vi "Test Viewer.vi"() -> ()   [LabVIEW 2016]
panel:
  out "XY Graph":cluster{"Y":dbl[], "Y":dbl[]}(graph)
  in  "channels":string[](array[string])=["Field (Resampled)", "U X (Resampled)", "U Y (Resampled)"]
  in  "group":string="p"
  in  "File Path Control":path=path "\\\\eden\\NHMFLDATA/Data/cell1daq/February_2017/021017/p002_021017.tdms"
  out "Waveform Graph":waveform(dbl)[](graph)
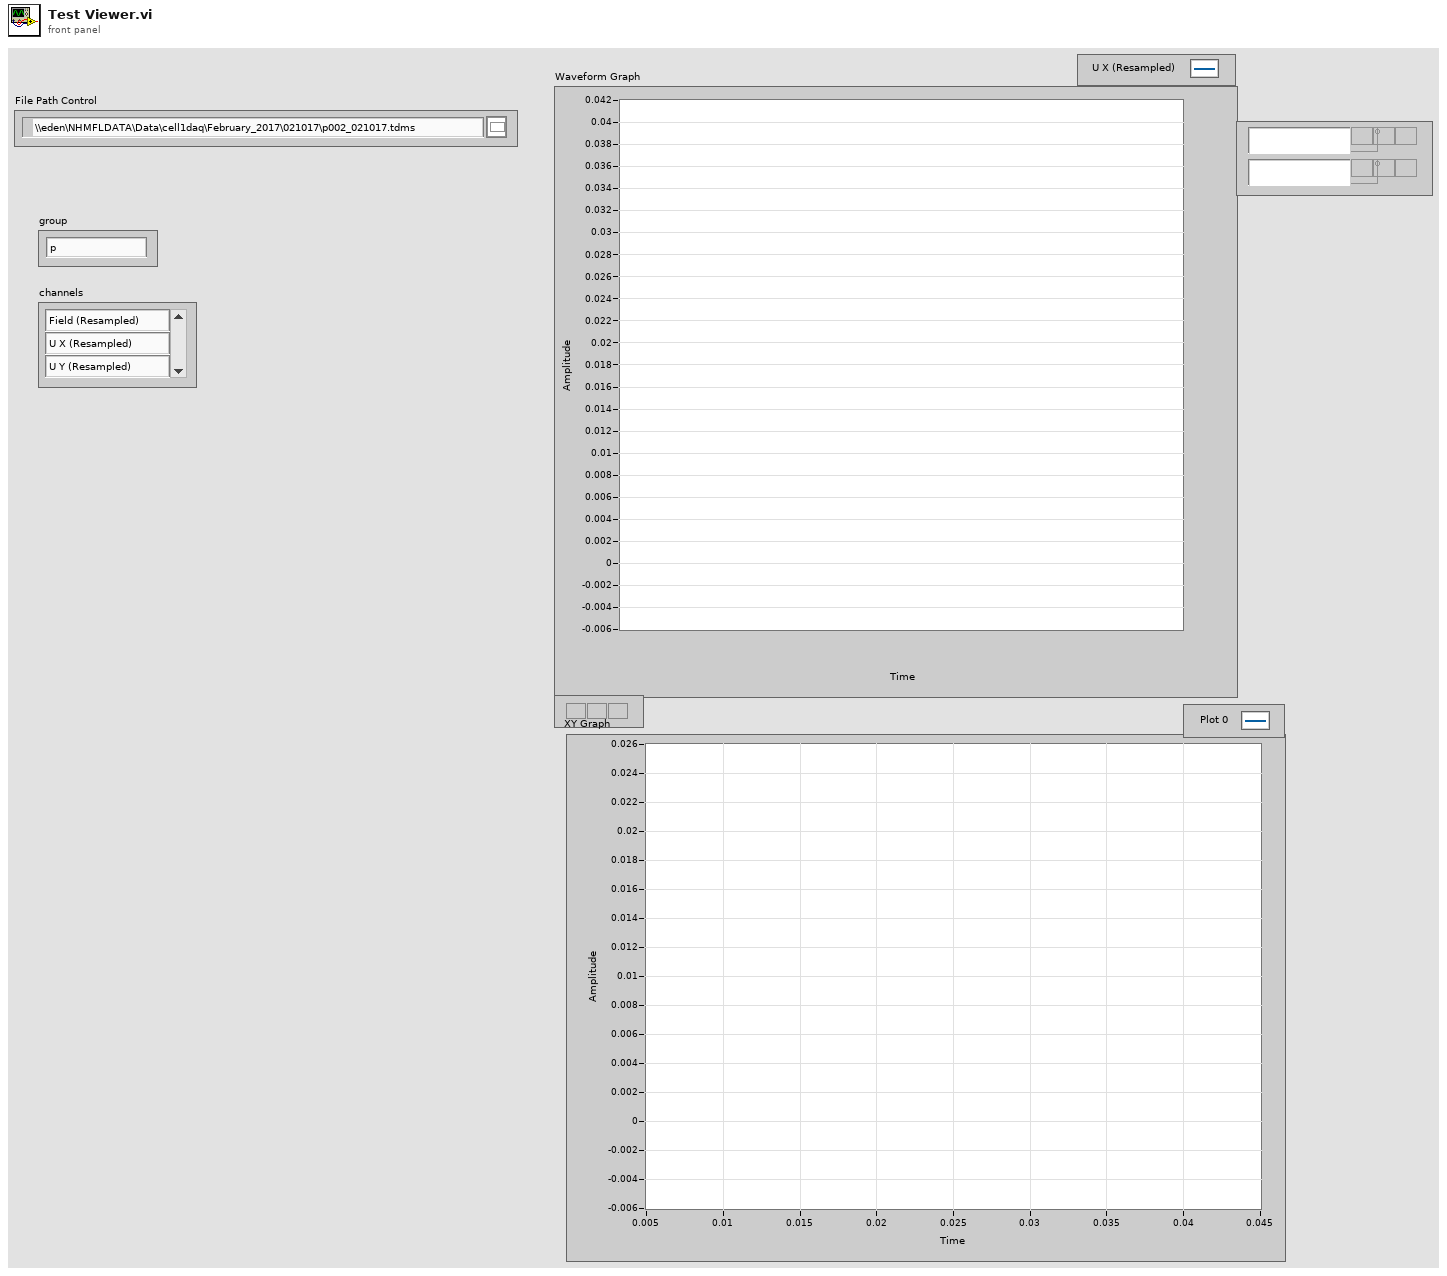
[diagram p1: front panel]
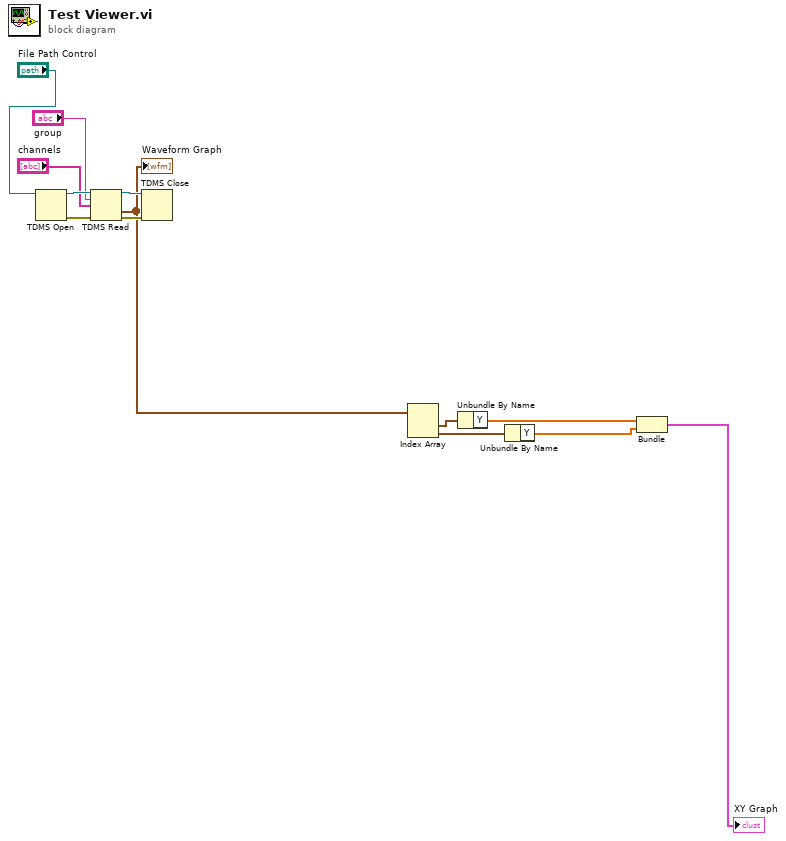
[diagram p0: block diagram]
diagram:
  n1 = TDMS Open(11:"File Path Control") -> (0:w10:errorcluster, 3:w13:refnum<k34>)  [unwired: 6 in]
  n2 = TDMS Read(0:w13, 5:"group", 7:"channels", 11:w10) -> (4:w12:refnum<k34>, 10:w6:waveform(dbl)[], 15:w11:errorcluster)  [unwired: 4 in, 3 out]
  "Waveform Graph" <- w6
  n3 = TDMS Close(8:w11, 11:w12) -> ()  [unwired: 2 out]
  n4 = Index Array(array=w6) -> (element #1=w5:waveform(dbl), element #2=w4:waveform(dbl))  [unwired: 2 in]
  n5 = Unbundle By Name(w5) -> ("Y"=w2:dbl[])
  n6 = Unbundle By Name(w4) -> ("Y"=w1:dbl[])
  n7 = Bundle("Y"=w2, "Y"=w1) -> (→"XY Graph":cluster{"Y":dbl[], "Y":dbl[]})  [unwired: 1 in]
